vi "STP.vi"(0 "System no.":i32=1 min=1 max=4 step=1, 2 "Affected axes?":string[](array[string]), 3 "All axes?":bool, 4 "Axis identifier?":bool=TRUE, 5 "error in":errorcluster) -> (19 "error out":errorcluster)   [LabVIEW 2020]
doc: "GCS 3.0\n=====\n\nSTP (Stop All Axes)\n\nDescription\nSTP stops all axes abruptly (i.e., with the maximum possible deceleration) and ends certain \ninternal processes (see Notes).\n\nFormat\nSTP\n\nArguments\nnone\n\nResponse\nnone\n\nNotes\nSTP ends the following internal processes:\n- Reference move\nIn contrast to STP, the HLT command (p. 19) can specifically stop one or more selected axes \nwhile taking account of the currently set motion parameters (e.g. the current deceleration ...).\nSTP does not cause a state transition in the drive state machine; for further details, see \"Drive \nState Machine\" (p. 101). \nIf some of the axes are not in the Operation enabled state when sending the STP command, STP \nis executed for all axes in the Operation enabled state.\n\nUser command level\nUSR\n\n\nGCS 2.0\n=====\n\nStops motion of specified axes (GCS2.x: Stops motion of all axes). To stop a referencing routine (REF, MNL, MPL) or fast scan routine (FSC, FSA etc.), or AutoZero procedure (ATZ), or wave generator run (WGO), use #24.vi. STP sets error code 10, call \"ERR?.vi\" to reset error after STP has been called.\n\nAnalog: All axes? = TRUE, Axis identifier = FALSE. STP does not set any error code.\nAll other systems: All axes? = TRUE, Axis identifier? = FALSE\n\nE-135: STP.vi stops motion of all axes caused by move commands (OSM, POL, SVA).\n\nE-517, E-518: STP.vi stops motion of all axes caused by move commands (MOV, MVR, GOH, SVA, SVR). Furthermore, it stops macros (MAC) and wave generator output (WGO).\n\nC-413, E-709, E-712, E-725, E-727, E-753, E-754: STP.vi stops motion of all axes caused by move commands (MOV, MVR, SVA, SVR), by the wave generator (WGO, if supported), by analog control input and autozero motion (ATZ).\n\nC-887, F-206, M-8X0: Only for GCS syntax version = GCS 2.0 or higher (check with CSV?.vi. If CSV?.vi is not supported, syntax version is GCS 1.0). For GCS 1.0, use STOP.vi instead."
panel:
  # "STP (Stop All Axes)\n\nSTP stops all axes abruptly (i.e., with the maximum possible deceleration) and ends certain internal processes (see Notes)."
  # "Stop"
  # "If all axes: use"
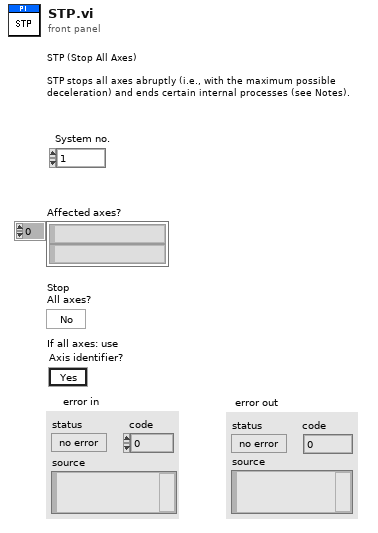
[diagram p1: front panel]
types:
  T1 = typedef "Syntax.ctl" = enum16{"GCS 1.0", "GCS 2.0", "GCS 3.0"}
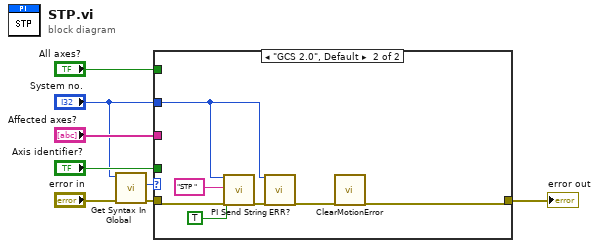
[diagram p0: block diagram]
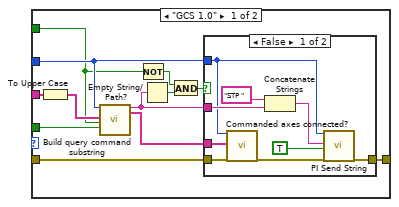
[diagram p2: hidden frame]
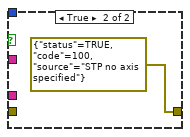
[diagram p3: hidden frame]
diagram:
  n1 = call "Get Syntax In Global.vi"("error in"="error in", "System no."="System no.") -> ("error out"=w2:errorcluster, "Syntax"=w1:T1)  [unwired: 8 in]
  n2 = case shown="\"GCS 2.0\", Default" w1 {
    tunnel: "Affected axes?" -> [w20 _]
    tunnel: "Axis identifier?" -> [w18 _]
    tunnel: "System no." -> [w17 w34]
    tunnel: "All axes?" -> [w15 _]
    tunnel: [w13 w31] -> w7
    tunnel: w2 -> [w11 w37]
    frame "GCS 1.0" {
      n3 = To Upper Case(1:w20) -> (0:w19:string[])
      n4 = call "Build query command substring.vi"("System no."=w17, "Axes to query in"=w19, "Query\nAll axes?"=w15, "For all axes: use\nAxis identifier?"=w18) -> ("Command substring"=w10:string, "Axes to query out"=w16:string[])  [unwired: 2 in, 12 out]
      n5 = Not(x=w15) -> (.not. x?=w14:bool)
      n6 = Empty String/Path?(string/path=w10) -> (empty?=w9:bool)
      n7 = And(x=w14, y=w9) -> (x .and. y?=w12:bool)
      n8 = case shown="False" w12 {
        tunnel: w10 -> [w26 _]
        tunnel: w17 -> [w25 _]
        tunnel: w16 -> [w24 _]
        tunnel: w11 -> [w22 _]
        tunnel: [w21 errorcluster {"status"=TRUE, "code"=100, "source"="STP no axis specified"} ("error out")] -> w13
        frame False {
          n9 = call "Commanded axes connected?.vi"("System no."=w25, "Commanded axes"=w24, "error in"=w22) -> ("error out"=w23:errorcluster)  [unwired: 1 in, 15 out]
          n10 = Concatenate Strings("STP ", w26) -> (w27:string)
          n11 = call "PI Send String.vi"("System no."=w25, "String to send"=w27, "Attach termination char.?"=TRUE ("Attach Linefeed?"), "error in"=w23) -> ("error out"=w21:errorcluster)  [unwired: 15 in]
        }
        frame True {
        }
      }
    }
    frame "GCS 2.0", Default {
      n12 = call "PI Send String.vi"("System no."=w34, "String to send"="STP ", "Attach termination char.?"=TRUE, "error in"=w37) -> ("error out"=w35:errorcluster)  [unwired: 15 in]
      n13 = call "ERR?.vi"("System no."=w34, "error in"=w35) -> ("error out"=w32:errorcluster)  [unwired: 17 out]
      n14 = call "ClearMotionError.vi"("error in (no error)"=w32) -> ("error out"=w31:errorcluster)  [unwired: 18 in]
    }
  }
  "error out" <- w7
